vi "p1.vi"() -> ()   [LabVIEW 2023, in "d2.lvlib"]
uses:
  d2.lvlib
  AOC/AOC.lvlib
panel:
  in  "Example":string="Game 1: 3 blue, 4 red; 1 red, 2 green, 6 blue; 2 green\nGame 2: 1 blue, 2 green; 3 green, 4 blue, 1 red; 1 green, 1 blue\nGame 3: 8 green, 6 blue, 20 red; 5 blue, 4 red, 13 green; 5 green, 1 red\nGame 4: 1 green, 3 red, 6 blue; 3 green, 6 red; 3 green, 15 blue, 14 red\nGame 5: 6 red, 1 blue, 3 green; 2 blue, 1 red, 2 green"
  in  "Example":bool
  out "Answer":i64=10624
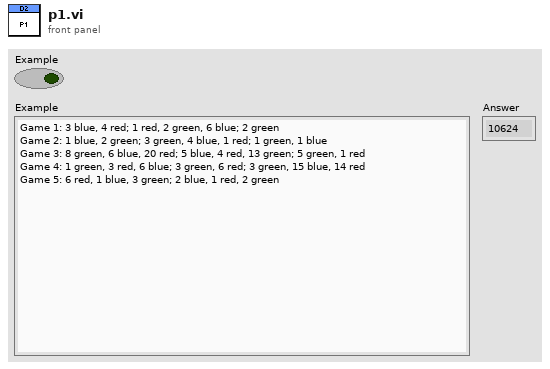
[diagram p1: front panel]
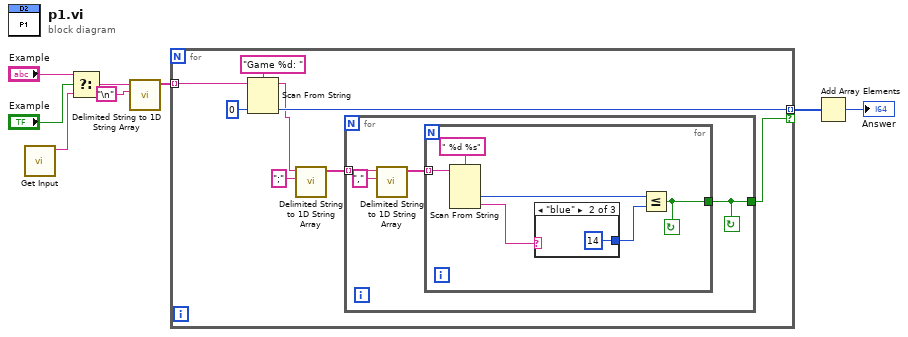
[diagram p0: block diagram]
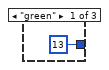
[diagram p2: hidden frame]
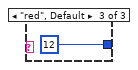
[diagram p3: hidden frame]
diagram:
  n1 = call "Get Input.vi"() -> ("Input"=w8:string)  [unwired: 11 in]
  n2 = Select(t="Example", s="Example", f=w8) -> (s? t:f=w7:string)
  n3 = call <vilib>:"Delimited String to 1D String Array.vi"("delimiter"="\n", "delimited string"=w7) -> ("string array"=w5:string[])  [unwired: 9 in]
  n4 = for {
    tunnel: w5 -> [w16] mode=indexing
    tunnel: [w14] -> w2 mode=indexing if=w10
    n5 = Scan From String(format string="Game %d: ", input string=w16, default 1=i64 0 ("default value 1")) -> (remaining string=w9:string, output 1=w14:i64)  [unwired: 2 in, 2 out]
    n6 = call <vilib>:"Delimited String to 1D String Array.vi"("delimiter"=";", "delimited string"=w9) -> ("string array"=w12:string[])  [unwired: 9 in]
    n7 = for {
      tunnel: w12 -> [w20] mode=indexing
      tunnel: [w17] -> w10
      stop <- w17 continue-if-true
      n8 = call <vilib>:"Delimited String to 1D String Array.vi"("delimiter"=",", "delimited string"=w20) -> ("string array"=w18:string[])  [unwired: 9 in]
      n9 = for {
        tunnel: w18 -> [w26] mode=indexing
        tunnel: [w21] -> w17
        stop <- w21 continue-if-true
        n10 = Scan From String(format string=" %d %s", input string=w26) -> (output 1=w22:i32, output 2=w24:string)  [unwired: 4 in, 3 out]
        n11 = case shown="\"blue\"" w24 {
          tunnel: [13 ("y") 14 ("y") 12 ("y")] -> w23
          frame "green" {
          }
          frame "blue" {
          }
          frame "red", Default {
          }
        }
        n12 = Less Or Equal?(x=w22, y=w23) -> (x <= y?=w21:bool)
      }
    }
  }
  n13 = Add Array Elements(numeric array=w2) -> (sum=→"Answer":i64)
